vi "addImageToScrollBar.vi"(8 "error in (no error)":errorcluster, 11 "ImageStreamViewer in":refnum<class "ImageStreamViewer.lvclass">) -> (0 "error out":errorcluster, 3 "ImageStreamViewer out":refnum<class "ImageStreamViewer.lvclass">)   [LabVIEW 2011, in "Views.lvlib" / "Camera.lvlib" / "ImageStreamViewer.lvclass"]
uses:
  ImageStreamViewer.lvclass
  ImageStreamViewer.lvclass/ImageStreamViewer.ctl
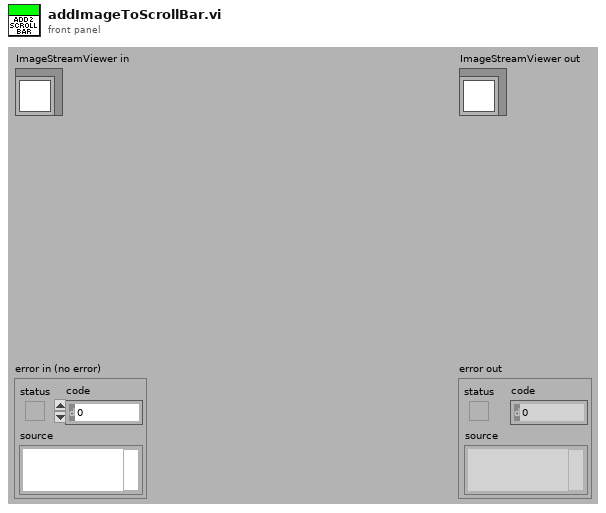
[diagram p1: front panel]
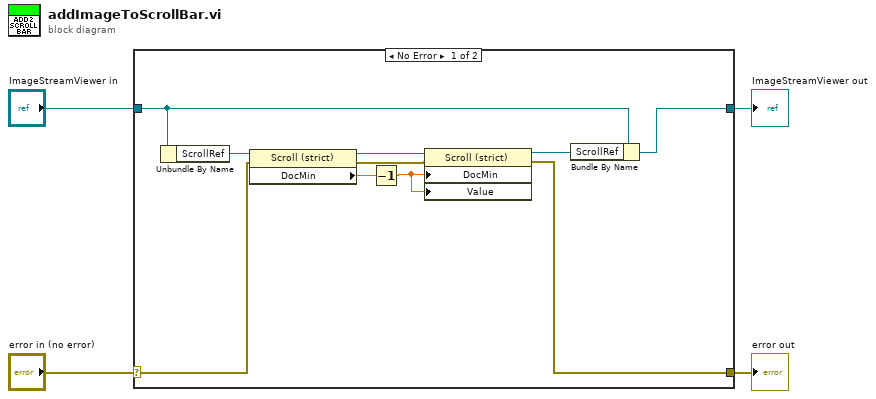
[diagram p0: block diagram]
diagram:
  n1 = case shown="No Error" "error in (no error)" {
    selector: "error in (no error)" -> [w13 w16]
    tunnel: [w5 w16] -> w3
    tunnel: [w7 w15] -> w1
    tunnel: "ImageStreamViewer in" -> [w8 w15]
    frame No Error {
      n2 = Unbundle By Name(w8) -> ("ScrollRef"=w14:refnum<vi>)
      n3 = property class="Scroll (strict)"(reference=w14, error in=w13) -> (reference out=w11:refnum<vi>, error out=w10:errorcluster, "DocMin"=w12:dbl)
      n4 = Decrement(x=w12) -> (x-1=w9:dbl)
      n5 = property class="Scroll (strict)"(reference=w11, error in=w10, "DocMin"=w9, "Value"=w9) -> (reference out=w6:refnum<vi>, error out=w5:errorcluster)
      n6 = Bundle By Name(cluster=w8, "ScrollRef"=w6) -> (w7:refnum<class "ImageStreamViewer.lvclass">)
    }
    frame Error {
    }
  }
  "error out" <- w3
  "ImageStreamViewer out" <- w1
